vi "SPIM control3d.vi"() -> ()   [LabVIEW 2012]
uses:
  Scanning Setting.vi
panel:
  out "Flash time":dbl
  in  "FLASH":bool
  out "Z-frequncy":dbl
  out "Z":dbl(slide)
  in  "Volum Scan":bool
  out "Trigger 4":dynamicdata(graph)=[{"t0"=timestamp(16448.7 s since 1904-01-01), "dt"=1e-05, "Y"=array[10000 elements], "attributes"=variant("NI_ChannelName"=variant(string "Triangle (Collected)"), "NI_ExpIsRelativeTime"=variant(bool TRUE), "NI_ExpStartTimeStamp"=variant(timestamp timestamp(3461934223.089551 s since 1904-01-01)), "NI_ExpTimeStamp"=variant(timestamp timestamp(3461934223.089551 s since 1904-01-01)), "NI_ExpXDimension"=variant(string "t"), "NI_OriginalChannelName"=variant(string "Triangle"))}, {"t0"=timestamp(16448.7 s since 1904-01-01), "dt"=1e-05, "Y"=array[10000 elements], "attributes"=variant("NI_ChannelName"=variant(string "Square (Collected)"), "NI_ExpIsRelativeTime"=variant(bool TRUE), "NI_ExpStartTimeStamp"=variant(timestamp timestamp(3461934223.089551 s since 1904-01-01)), "NI_ExpTimeStamp"=variant(timestamp timestamp(3461934223.089551 s since 1904-01-01)), "NI_ExpXDimension"=variant(string "t"), "NI_OriginalChannelName"=variant(string "Square"))}, {"t0"=timestamp(16448.7 s since 1904-01-01), "dt"=1e-05, "Y"=array[10000 elements], "attributes"=variant("NI_ChannelName"=variant(string "Square (Collected)"), "NI_ExpIsRelativeTime"=variant(bool TRUE), "NI_ExpStartTimeStamp"=variant(timestamp timestamp(3461934223.0885506 s since 1904-01-01)), "NI_ExpTimeStamp"=variant(timestamp timestamp(3461934223.0885506 s since 1904-01-01)), "NI_ExpXDimension"=variant(string "t"), "NI_OriginalChannelName"=variant(string "Square"))}]
  out "Trigger 3":dynamicdata(graph)=[{"t0"=timestamp(16448.7 s since 1904-01-01), "dt"=1e-05, "Y"=array[10000 elements], "attributes"=variant("NI_ChannelName"=variant(string "Triangle (Collected)"), "NI_ExpIsRelativeTime"=variant(bool TRUE), "NI_ExpStartTimeStamp"=variant(timestamp timestamp(3461934223.089551 s since 1904-01-01)), "NI_ExpTimeStamp"=variant(timestamp timestamp(3461934223.089551 s since 1904-01-01)), "NI_ExpXDimension"=variant(string "t"), "NI_OriginalChannelName"=variant(string "Triangle"))}, {"t0"=timestamp(16448.7 s since 1904-01-01), "dt"=1e-05, "Y"=array[10000 elements], "attributes"=variant("NI_ChannelName"=variant(string "Square (Collected)"), "NI_ExpIsRelativeTime"=variant(bool TRUE), "NI_ExpStartTimeStamp"=variant(timestamp timestamp(3461934223.089551 s since 1904-01-01)), "NI_ExpTimeStamp"=variant(timestamp timestamp(3461934223.089551 s since 1904-01-01)), "NI_ExpXDimension"=variant(string "t"), "NI_OriginalChannelName"=variant(string "Square"))}, {"t0"=timestamp(16448.7 s since 1904-01-01), "dt"=1e-05, "Y"=array[10000 elements], "attributes"=variant("NI_ChannelName"=variant(string "Square (Collected)"), "NI_ExpIsRelativeTime"=variant(bool TRUE), "NI_ExpStartTimeStamp"=variant(timestamp timestamp(3461934223.0885506 s since 1904-01-01)), "NI_ExpTimeStamp"=variant(timestamp timestamp(3461934223.0885506 s since 1904-01-01)), "NI_ExpXDimension"=variant(string "t"), "NI_OriginalChannelName"=variant(string "Square"))}]
  out "Trigger 2":dynamicdata(graph)=[{"t0"=timestamp(16448.7 s since 1904-01-01), "dt"=1e-05, "Y"=array[10000 elements], "attributes"=variant("NI_ChannelName"=variant(string "Triangle (Collected)"), "NI_ExpIsRelativeTime"=variant(bool TRUE), "NI_ExpStartTimeStamp"=variant(timestamp timestamp(3461934223.089551 s since 1904-01-01)), "NI_ExpTimeStamp"=variant(timestamp timestamp(3461934223.089551 s since 1904-01-01)), "NI_ExpXDimension"=variant(string "t"), "NI_OriginalChannelName"=variant(string "Triangle"))}, {"t0"=timestamp(16448.7 s since 1904-01-01), "dt"=1e-05, "Y"=array[10000 elements], "attributes"=variant("NI_ChannelName"=variant(string "Square (Collected)"), "NI_ExpIsRelativeTime"=variant(bool TRUE), "NI_ExpStartTimeStamp"=variant(timestamp timestamp(3461934223.089551 s since 1904-01-01)), "NI_ExpTimeStamp"=variant(timestamp timestamp(3461934223.089551 s since 1904-01-01)), "NI_ExpXDimension"=variant(string "t"), "NI_OriginalChannelName"=variant(string "Square"))}, {"t0"=timestamp(16448.7 s since 1904-01-01), "dt"=1e-05, "Y"=array[10000 elements], "attributes"=variant("NI_ChannelName"=variant(string "Square (Collected)"), "NI_ExpIsRelativeTime"=variant(bool TRUE), "NI_ExpStartTimeStamp"=variant(timestamp timestamp(3461934223.0885506 s since 1904-01-01)), "NI_ExpTimeStamp"=variant(timestamp timestamp(3461934223.0885506 s since 1904-01-01)), "NI_ExpXDimension"=variant(string "t"), "NI_OriginalChannelName"=variant(string "Square"))}]
  in  "1 Slice":bool
  in  "Structual":bool
  in  "Funcational":bool
  out "Peizo Voltage":dbl
  out "Peizo Location":dbl
  out "Z-Offset":dbl
  out "Scan Signal 2":cluster{"Y":dbl[], "Y":dbl[]}[](graph)
  out "Trigger":dynamicdata(graph)=[{"t0"=timestamp(16448.7 s since 1904-01-01), "dt"=1e-05, "Y"=array[10000 elements], "attributes"=variant("NI_ChannelName"=variant(string "Triangle (Collected)"), "NI_ExpIsRelativeTime"=variant(bool TRUE), "NI_ExpStartTimeStamp"=variant(timestamp timestamp(3461934223.089551 s since 1904-01-01)), "NI_ExpTimeStamp"=variant(timestamp timestamp(3461934223.089551 s since 1904-01-01)), "NI_ExpXDimension"=variant(string "t"), "NI_OriginalChannelName"=variant(string "Triangle"))}, {"t0"=timestamp(16448.7 s since 1904-01-01), "dt"=1e-05, "Y"=array[10000 elements], "attributes"=variant("NI_ChannelName"=variant(string "Square (Collected)"), "NI_ExpIsRelativeTime"=variant(bool TRUE), "NI_ExpStartTimeStamp"=variant(timestamp timestamp(3461934223.089551 s since 1904-01-01)), "NI_ExpTimeStamp"=variant(timestamp timestamp(3461934223.089551 s since 1904-01-01)), "NI_ExpXDimension"=variant(string "t"), "NI_OriginalChannelName"=variant(string "Square"))}, {"t0"=timestamp(16448.7 s since 1904-01-01), "dt"=1e-05, "Y"=array[10000 elements], "attributes"=variant("NI_ChannelName"=variant(string "Square (Collected)"), "NI_ExpIsRelativeTime"=variant(bool TRUE), "NI_ExpStartTimeStamp"=variant(timestamp timestamp(3461934223.0885506 s since 1904-01-01)), "NI_ExpTimeStamp"=variant(timestamp timestamp(3461934223.0885506 s since 1904-01-01)), "NI_ExpXDimension"=variant(string "t"), "NI_OriginalChannelName"=variant(string "Square"))}]
  out "Scan Signal":cluster{"Y":dbl[], "Y":dbl[]}[](graph)
  out "Error Out":errorcluster={"status"=TRUE, "code"=-200561, "source"="SPIM control.vi:Instance:14:1<append>\n<B>Data: </B>-10.007205\n<B>Specified Range Minimum: </B>-10.0\n<B>Specified Range Maximum: </B> 10.0\n\n<B>Task Name: </B>_unnamedTask<30>"}
  in  "Scanner":bool
  in  "Setting":bool
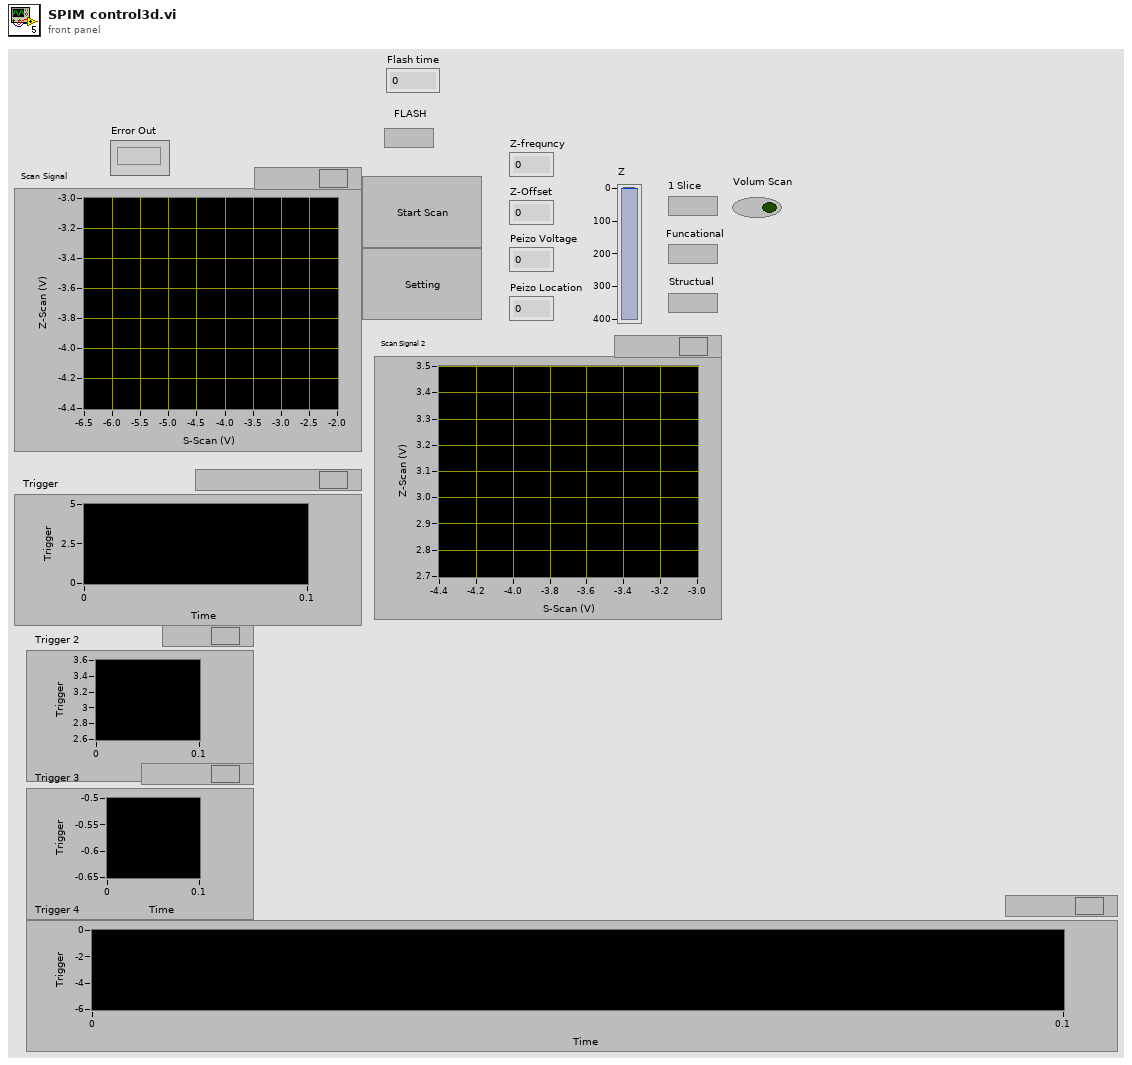
[diagram p1: front panel]
types:
  T1 = enum8{"Enabled", "Disabled", "Disabled and Grayed Out"}
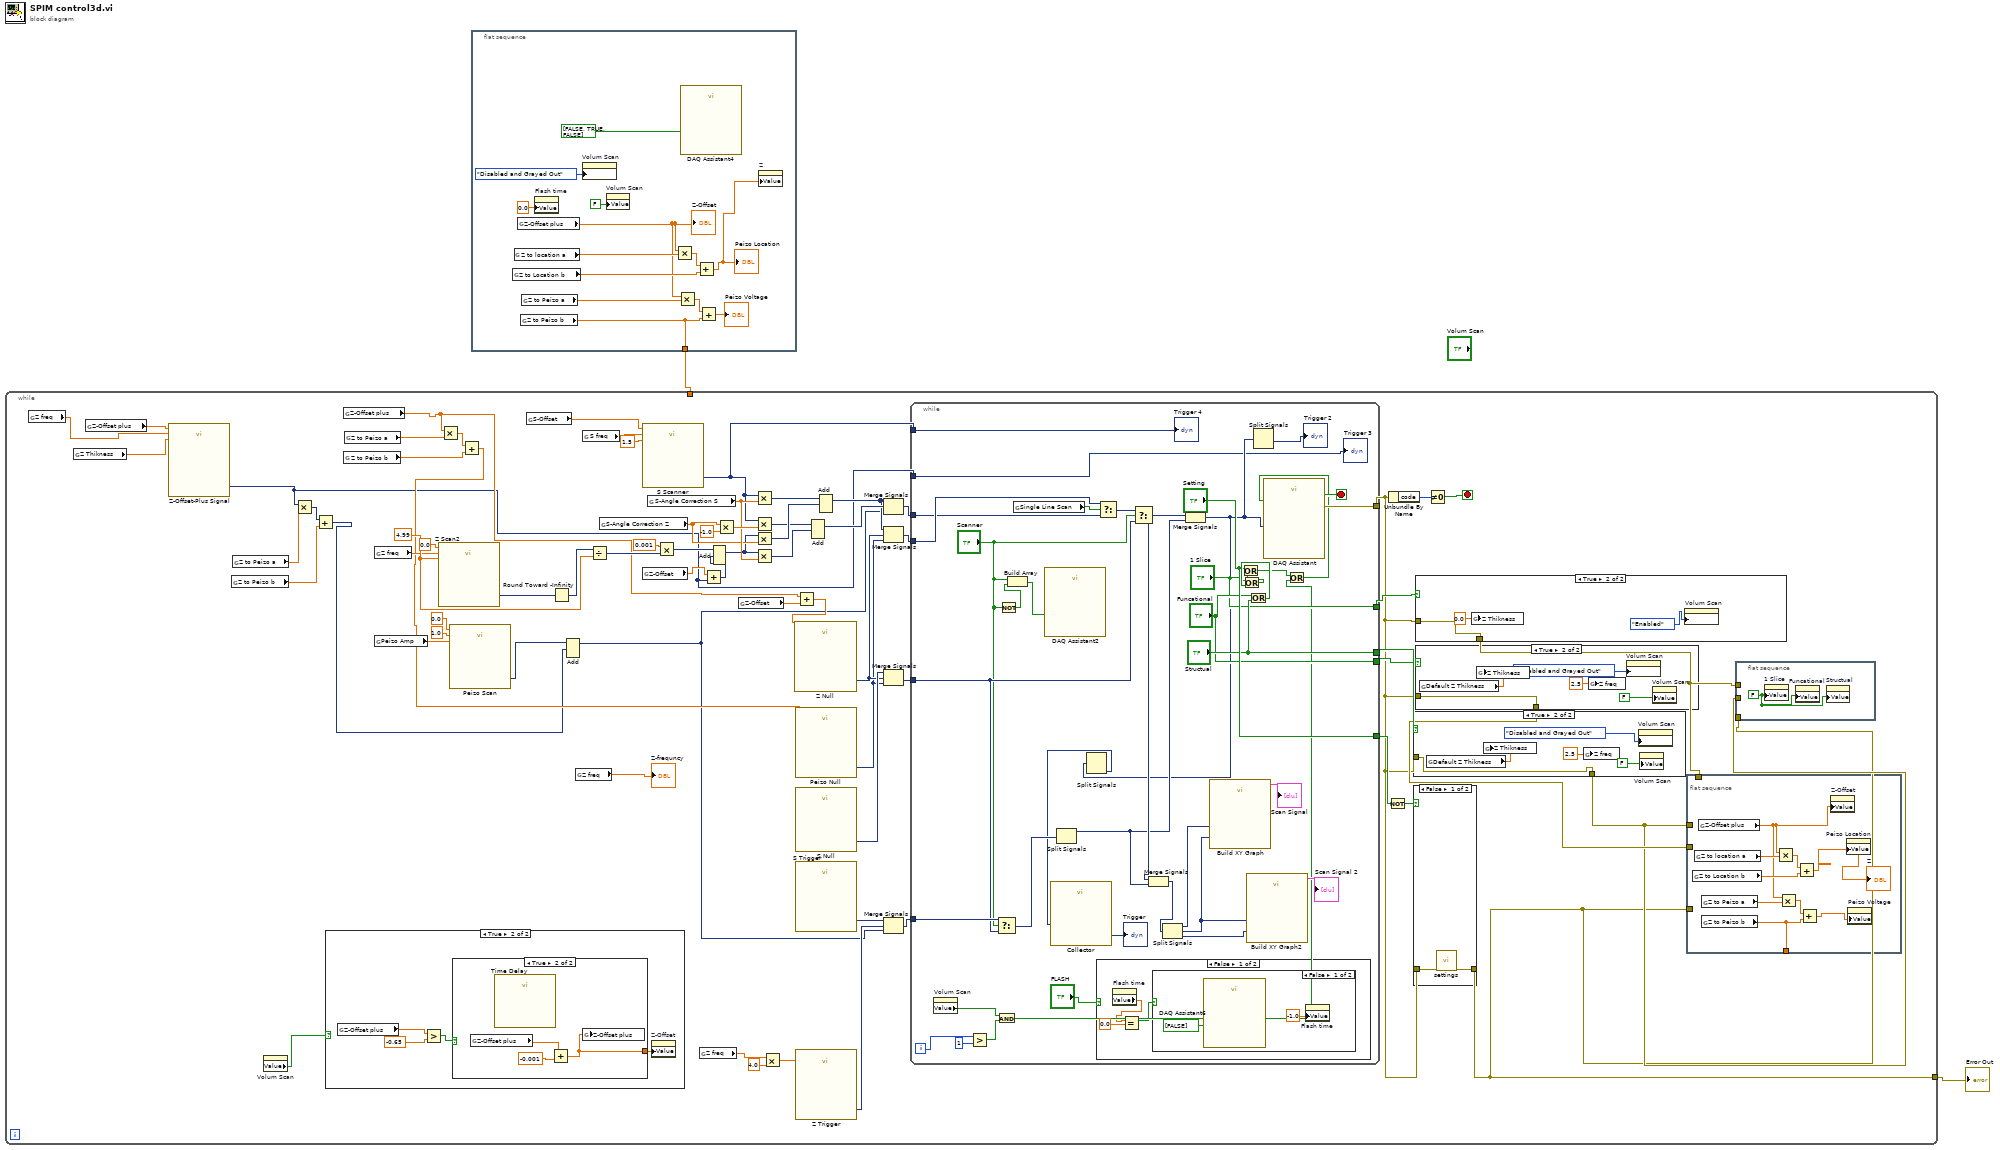
[diagram p0: block diagram]
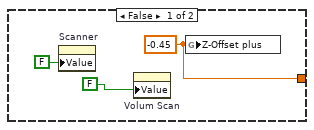
[diagram p3: hidden frame]
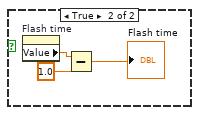
[diagram p8: hidden frame]
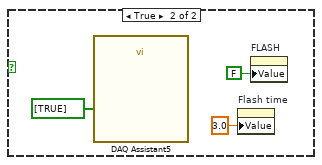
[diagram p9: hidden frame]
diagram:
  n1 = while {
    tunnel: [w8] -> w1
    tunnel: w2 -> [_]
    stop <- w47 stop-if-true
    w45 = 4.99 ("Amplitude")
    n2 = global read "Scanning Setting.vi" "Z freq"() -> (w17:dbl)
    n3 = global read "Scanning Setting.vi" "Z Thikness"() -> (w18:dbl)
    n4 = global read "Scanning Setting.vi" "Z-Offset plus"() -> (w26:dbl)
    n5 = call "Z-Offset-Plus Signal"("Offset"=w26, "Frequency"=w17, "Amplitude"=w18) -> ("Triangle"=w6:dynamicdata)  [unwired: 11 in, 1 out]
    n6 = global read "Scanning Setting.vi" "Z to Peizo b"() -> (w25:dbl)
    n7 = global read "Scanning Setting.vi" "Z to Peizo a"() -> (w24:dbl)
    n8 = property on="Volum Scan" class="Bool (strict)"() -> ("Value"=w4:bool)  [unwired: 2 in, 2 out]
    n9 = Multiply(x=w6, y=w24) -> (x*y=w23:dynamicdata)
    n10 = Add(x=w23, y=w25) -> (x+y=w21:dynamicdata)
    n11 = case shown="True" w4 {
      frame False {
      }
      frame True {
        n12 = global read "Scanning Setting.vi" "Z-Offset plus"() -> (w76:dbl)
        n13 = Greater?(x=w76, y=-0.65) -> (0:w77:bool)
        n14 = case shown="True" w77 {
          tunnel: [w79 w81] -> w74
          frame False {
            w79 = -0.45 ("Z-Offset plus")
            n15 = property on="Scanner" class="Bool (strict)"("Value"=FALSE ("Scanner")) -> ()  [unwired: 2 in, 2 out]
            n16 = property on="Volum Scan" class="Bool (strict)"("Value"=FALSE) -> ()  [unwired: 2 in, 2 out]
            n17 = global write "Scanning Setting.vi" "Z-Offset plus"(w79) -> ()
          }
          frame True {
            n18 = global read "Scanning Setting.vi" "Z-Offset plus"() -> (w82:dbl)
            n19 = call "Time Delay"() -> ()  [unwired: 11 in, 1 out]
            n20 = Add(x=w82, y=-0.001) -> (x+y=w81:dbl)
            n21 = global write "Scanning Setting.vi" "Z-Offset plus"(w81) -> ()
          }
        }
        n22 = property on="Z-Offset" class="DigNum (strict)"("Value"=w74) -> ()  [unwired: 2 in, 2 out]
      }
    }
    n23 = global read "Scanning Setting.vi" "Z-Offset plus"() -> (w27:dbl)
    n24 = global read "Scanning Setting.vi" "Z to Peizo b"() -> (w29:dbl)
    n25 = global read "Scanning Setting.vi" "Z to Peizo a"() -> (w30:dbl)
    n26 = global read "Scanning Setting.vi" "Peizo Amp"() -> (w37:dbl)
    n27 = global read "Scanning Setting.vi" "Z freq"() -> (w38:dbl)
    n28 = call "Z Scan2"("Offset"=0.0, "Frequency"=w38, "Amplitude"=w45) -> ("Triangle"=w42:dynamicdata)  [unwired: 11 in, 1 out]
    n29 = Multiply(x=w27, y=w30) -> (x*y=w31:dbl)
    n30 = call "Peizo Scan"("Offset"=0.0, "Frequency"=1.0, "Amplitude"=w37) -> ("Sine"=w22:dynamicdata)  [unwired: 11 in, 1 out]
    n31 = Add(x=w31, y=w29) -> (x+y=w28:dbl)
    n32 = global read "Scanning Setting.vi" "S-Offset"() -> (w61:dbl)
    n33 = Round Toward -Infinity(1:w42) -> (0:w43:dynamicdata)
    n34 = Add(1:w21, 2:w22) -> (0:w20:dynamicdata)  [unwired: 1 in, 1 out]
    n35 = global read "Scanning Setting.vi" "Z freq"() -> (→"Z-frequncy":dbl)
    n36 = global read "Scanning Setting.vi" "S freq"() -> (w62:dbl)
    n37 = Divide(x=w43, y=w45) -> (x/y=w46:dynamicdata)
    n38 = global read "Scanning Setting.vi" "S-Angle Correction Z"() -> (w59:dbl)
    n39 = call "S Scanner"("Offset"=w61, "Frequency"=w62, "Amplitude"=1.5) -> ("Triangle"=w5:dynamicdata)  [unwired: 11 in, 1 out]
    n40 = global read "Scanning Setting.vi" "Z-Offset"() -> (w35:dbl)
    n41 = global read "Scanning Setting.vi" "S-Angle Correction S"() -> (w60:dbl)
    n42 = Multiply(x=0.001, y=w46) -> (x*y=w41:dynamicdata)
    n43 = global read "Scanning Setting.vi" "Z freq"() -> (w50:dbl)
    n44 = Add(x=w35, y=w6) -> (x+y=w34:dynamicdata)
    n45 = Add(1:w34, 2:w41) -> (0:w40:dynamicdata)  [unwired: 1 in, 1 out]
    n46 = Multiply(x=w59, y=-1.0) -> (x*y=w65:dbl)
    n47 = global read "Scanning Setting.vi" "Z-Offset"() -> (w33:dbl)
    n48 = Multiply(x=w5, y=w60) -> (x*y=w68:dynamicdata)
    n49 = Multiply(x=w5, y=w65) -> (x*y=w66:dynamicdata)
    n50 = Multiply(x=w40, y=w59) -> (x*y=w69:dynamicdata)
    n51 = Multiply(x=w40, y=w60) -> (x*y=w67:dynamicdata)
    n52 = Multiply(x=w50, y=4.0) -> (x*y=w51:dbl)
    n53 = call "Peizo Null"("Offset"=w28) -> ("Square"=w39:dynamicdata)  [unwired: 13 in, 1 out]
    n54 = call "S Null"() -> ("Triangle"=w73:dynamicdata)  [unwired: 14 in, 1 out]
    n55 = call "S Trigger"() -> ("Square"=w55:dynamicdata)  [unwired: 14 in, 1 out]
    n56 = call "Z Trigger"("Frequency"=w51) -> ("Square"=w54:dynamicdata)  [unwired: 13 in, 1 out]
    n57 = Add(x=w27, y=w33) -> (x+y=w32:dbl)
    n58 = call "Z Null"("Offset"=w32) -> ("Square"=w58:dynamicdata)  [unwired: 13 in, 1 out]
    n59 = Add(1:w67, 2:w66) -> (0:w63:dynamicdata)  [unwired: 1 in, 1 out]
    n60 = Add(1:w69, 2:w68) -> (0:w57:dynamicdata)  [unwired: 1 in, 1 out]
    n61 = Merge Signals(w57, w63, w20) -> (w72:dynamicdata)
    n62 = Merge Signals(w57, w58, w39) -> (w56:dynamicdata)
    n63 = Merge Signals(w73, w58, w39) -> (w71:dynamicdata)
    n64 = Merge Signals(w55, w54, w20) -> (w53:dynamicdata)
    n65 = while {
      tunnel: w72 -> [w147]
      tunnel: w71 -> [w142]
      tunnel: [w150] -> w7
      tunnel: w56 -> [w149]
      tunnel: w53 -> [w143]
      tunnel: ["Setting"] -> w15
      tunnel: ["Structual"] -> w14
      tunnel: ["Funcational"] -> w13
      tunnel: ["1 Slice"] -> w12
      tunnel: w6 -> [w122]
      tunnel: w5 -> [w121]
      i -> [w120]
      stop <- w152 stop-if-true
      n66 = property on="Volum Scan" class="Bool (strict)"() -> ("Value"=w117:bool)  [unwired: 2 in, 2 out]
      n67 = Greater?(x=w120, y=1) -> (0:w118:bool)
      n68 = Select(t=w143, s="Scanner", f=w142) -> (s? t:f=w137:dynamicdata)
      n69 = And(x=w117, y=w118) -> (x .and. y?=w114:bool)
      n70 = Not(x="Scanner") -> (.not. x?=w126:bool)
      n71 = Build Array("Scanner", w126) -> (w127:bool[])
      n72 = global read "Scanning Setting.vi" "Single Line Scan"() -> (w148:bool)
      n73 = call "DAQ Assistant2"("data"=w127) -> ()  [unwired: 17 in, 2 out]
      n74 = Split Signals(w137) -> (w134:dynamicdata)  [unwired: 3 in, 2 out]
      n75 = case shown="False" "FLASH" {
        frame False {
          n76 = property on="Flash time" class="DigNum (strict)"() -> ("Value"=w153:dbl)  [unwired: 2 in, 2 out]
          n77 = Equal?(x=w153, y=0.0) -> (x = y?=w154:bool)
          n78 = case shown="False" w154 {
            frame False {
              n79 = call "DAQ Assistant6"("data"=bool[] [FALSE]) -> ()  [unwired: 17 in, 2 out]
              n80 = property on="Flash time" class="DigNum (strict)"("Value"=-1.0 ("Flash time")) -> ()  [unwired: 2 in, 2 out]
            }
            frame True {
              n81 = property on="Flash time" class="DigNum (strict)"() -> ("Value"=w160:dbl)  [unwired: 2 in, 2 out]
              n82 = Subtract(x=w160, y=1.0) -> (x-y=→"Flash time":dbl)
            }
          }
        }
        frame True {
          n83 = call "DAQ Assistant5"("data"=bool[] [TRUE]) -> ()  [unwired: 17 in, 2 out]
          n84 = property on="Flash time" class="DigNum (strict)"("Value"=3.0 ("Flash time")) -> ()  [unwired: 2 in, 2 out]
          n85 = property on="FLASH" class="Bool (strict)"("Value"=FALSE ("FLASH")) -> ()  [unwired: 2 in, 2 out]
        }
      }
      n86 = Select(t=w149, s=w148, f=w147) -> (s? t:f=w146:dynamicdata)
      n87 = Select(t=w146, s="Scanner", f=w142) -> (s? t:f=w145:dynamicdata)
      n88 = Merge Signals(w145, w134) -> (w135:dynamicdata)
      n89 = Split Signals(w135) -> (w139:dynamicdata, w140:dynamicdata, w138:dynamicdata)  [unwired: 3 in]
      n90 = Merge Signals(w145, w134) -> (w124:dynamicdata)
      n91 = Split Signals(w124) -> (w136:dynamicdata)  [unwired: 4 in, 3 out]
      n92 = call "Collector"("Signals"=w136) -> ("Collected Signals"=→"Trigger":dynamicdata)  [unwired: 9 in, 1 out]
      n93 = call "Build XY Graph"("Y Input"=w140, "X Input"=w139) -> ("XY Graph"=→"Scan Signal":cluster{"Y":dbl[], "Y":dbl[]}[])  [unwired: 3 in, 6 out]
      n94 = call "Build XY Graph2"("Y Input"=w138, "X Input"=w140) -> ("XY Graph"=→"Scan Signal 2":cluster{"Y":dbl[], "Y":dbl[]}[])  [unwired: 3 in, 6 out]
      n95 = Or(x="Funcational", y="Structual") -> (x .or. y?=w133:bool)
      n96 = Or(x="1 Slice", y=w133) -> (x .or. y?=w132:bool)
      n97 = Or(x="Setting", y=w132) -> (x .or. y?=w115:bool)
      n98 = Split Signals(w124) -> (→"Trigger 2":dynamicdata)  [unwired: 4 in, 3 out]
      n99 = Or(x=w115, y=w114) -> (x .or. y?=w116:bool)
      n100 = call "DAQ Assistant"("data"=w124, "stop (F)"=w116) -> ("stopped"=w152:bool, "error out"=w150:errorcluster)  [unwired: 15 in, 1 out]
      "Trigger 3" <- w122
      "Trigger 4" <- w121
    }
    n101 = Not(x=w15) -> (.not. x?=w16:bool)
    n102 = Unbundle By Name(w7) -> ("code"=w48:i32)
    n103 = case shown="True" w14 {
      tunnel: w7 -> [w95 w98]
      tunnel: [w95 w98] -> w9
      frame False {
      }
      frame True {
        n104 = global read "Scanning Setting.vi" "Default Z Thikness"() -> (w100:dbl)
        n105 = global write "Scanning Setting.vi" "Z Thikness"(w100) -> ()
        n106 = global write "Scanning Setting.vi" "Z freq"(2.5 ("Z freq")) -> ()
        n107 = property on="Volum Scan" class="Bool (strict)"("DisabledEnum"=T1."Disabled and Grayed Out" ("Disabled")) -> ()  [unwired: 2 in, 2 out]
        n108 = property on="Volum Scan" class="Bool (strict)"("Value"=FALSE ("Volum Scan")) -> ()  [unwired: 2 in, 2 out]
      }
    }
    n109 = case shown="False" w16 {
      tunnel: [w110 w112] -> w8
      tunnel: w7 -> [w111 w112]
      frame False {
        n110 = call "settings.vi"("Error In"=w111) -> ("Error Out"=w110:errorcluster)  [unwired: 10 in]
      }
      frame True {
      }
    }
    n111 = case shown="True" w12 {
      tunnel: w7 -> [w85 w87]
      tunnel: [w85 w87] -> w10
      frame False {
      }
      frame True {
        n112 = global write "Scanning Setting.vi" "Z Thikness"(0.0 ("Z Thikness")) -> ()
        n113 = property on="Volum Scan" class="Bool (strict)"("DisabledEnum"=T1."Enabled" ("Disabled")) -> ()  [unwired: 2 in, 2 out]
      }
    }
    n114 = case shown="True" w13 {
      tunnel: w7 -> [w89 w92]
      tunnel: [w89 w92] -> w11
      frame False {
      }
      frame True {
        n115 = global read "Scanning Setting.vi" "Default Z Thikness"() -> (w94:dbl)
        n116 = global write "Scanning Setting.vi" "Z Thikness"(w94) -> ()
        n117 = global write "Scanning Setting.vi" "Z freq"(2.5 ("Z freq")) -> ()
        n118 = property on="Volum Scan" class="Bool (strict)"("DisabledEnum"=T1."Disabled and Grayed Out" ("Disabled")) -> ()  [unwired: 2 in, 2 out]
        n119 = property on="Volum Scan" class="Bool (strict)"("Value"=FALSE ("Volum Scan")) -> ()  [unwired: 2 in, 2 out]
      }
    }
    n120 = Not Equal To 0?(x=w48) -> (x != 0?=w47:bool)
    n121 = flat-sequence {
      tunnel: [w104] -> _
      tunnel: w8 -> [_]
      tunnel: w9 -> [_]
      tunnel: w11 -> [_]
      tunnel: w10 -> [_]
      frame #0 {
        n122 = global read "Scanning Setting.vi" "Z to Location b"() -> (w107:dbl)
        n123 = global read "Scanning Setting.vi" "Z to location a"() -> (w109:dbl)
        n124 = global read "Scanning Setting.vi" "Z-Offset plus"() -> (w103:dbl)
        n125 = global read "Scanning Setting.vi" "Z to Peizo b"() -> (w104:dbl)
        n126 = global read "Scanning Setting.vi" "Z to Peizo a"() -> (w105:dbl)
        n127 = Multiply(x=w103, y=w109) -> (x*y=w108:dbl)
        n128 = Multiply(x=w103, y=w105) -> (x*y=w106:dbl)
        n129 = Add(x=w108, y=w107) -> (x+y=w101:dbl)
        "Z" <- w101
        n130 = Add(x=w106, y=w104) -> (x+y=w102:dbl)
        n131 = property on="Z-Offset" class="DigNum (strict)"("Value"=w103) -> ()  [unwired: 2 in, 2 out]
        n132 = property on="Peizo Location" class="DigNum (strict)"("Value"=w101) -> ()  [unwired: 2 in, 2 out]
        n133 = property on="Peizo Voltage" class="DigNum (strict)"("Value"=w102) -> ()  [unwired: 2 in, 2 out]
      }
    }
    n134 = flat-sequence {
      tunnel: w10 -> [_]
      tunnel: w9 -> [_]
      tunnel: w8 -> [_]
      frame #0 {
        w84 = FALSE ("1 Slice")
        n135 = property on="1 Slice" class="Bool (strict)"("Value"=w84) -> ()  [unwired: 2 in, 2 out]
        n136 = property on="Funcational" class="Bool (strict)"("Value"=w84) -> ()  [unwired: 2 in, 2 out]
        n137 = property on="Structual" class="Bool (strict)"("Value"=w84) -> ()  [unwired: 2 in, 2 out]
      }
    }
  }
  "Error Out" <- w1
  n138 = flat-sequence {
    tunnel: [w169] -> w2
    frame #0 {
      n139 = global read "Scanning Setting.vi" "Z to Location b"() -> (w174:dbl)
      n140 = global read "Scanning Setting.vi" "Z to location a"() -> (w176:dbl)
      n141 = global read "Scanning Setting.vi" "Z-Offset plus"() -> (w170:dbl)
      "Z-Offset" <- w170
      n142 = global read "Scanning Setting.vi" "Z to Peizo b"() -> (w169:dbl)
      n143 = global read "Scanning Setting.vi" "Z to Peizo a"() -> (w172:dbl)
      n144 = property on="Flash time" class="DigNum (strict)"("Value"=0.0 ("Flash time")) -> ()  [unwired: 2 in, 2 out]
      n145 = property on="Volum Scan" class="Bool (strict)"("DisabledEnum"=T1."Disabled and Grayed Out" ("Disabled")) -> ()  [unwired: 2 in, 2 out]
      n146 = property on="Volum Scan" class="Bool (strict)"("Value"=FALSE ("Volum Scan")) -> ()  [unwired: 2 in, 2 out]
      n147 = Multiply(x=w170, y=w176) -> (x*y=w175:dbl)
      n148 = Multiply(x=w170, y=w172) -> (x*y=w173:dbl)
      n149 = call "DAQ Assistant4"("data"=bool[] [FALSE, TRUE, FALSE]) -> ()  [unwired: 17 in, 2 out]
      n150 = Add(x=w175, y=w174) -> (x+y=w165:dbl)
      "Peizo Location" <- w165
      n151 = Add(x=w173, y=w169) -> (x+y=→"Peizo Voltage":dbl)
      n152 = property on="Z" class="Slide (strict)"("Value"=w165) -> ()  [unwired: 2 in, 2 out]
    }
  }
